vi "GetDnetStrings.vi"() -> ()   [LabVIEW 2011]
uses:
  Controls/Device Cluster.ctl
  <vilib>/Utility/file.llb/Read From Spreadsheet File (string).vi
  GlobalVariables.vi
panel:
  in  "Device Cluster":T1={"Dnet"="", "Node"=0, "Type"="", "ID Number"=0, "SCCM"=0.0, "FullScale"=0.0, "Input Bytes"=0, "Output Bytes"=0, "Input Start Location"=0, "Output Start Location"=0, "Enabled"=TRUE, "Bytes"=[0, 0, 0]}
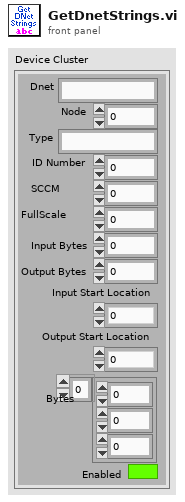
[diagram p1: front panel]
types:
  T1 = typedef "Device Cluster.ctl" = cluster{"Dnet":string, "Node":i32, "Type":string, "ID Number":u8, "SCCM":dbl, "FullScale":dbl, "Input Bytes":i32, "Output Bytes":i32, "Input Start Location":i32, "Output Start Location":i32, "Enabled":bool, "Bytes":u8[]}
  T2 = cluster{"all rows[0]":string, "all rows[1]":string, "all rows[2]":string, "all rows[3]":string, "all rows[4]":string, "all rows[5]":string, "all rows[6]":string, "all rows[7]":string, "all rows[8]":string, "all rows[9]":string}
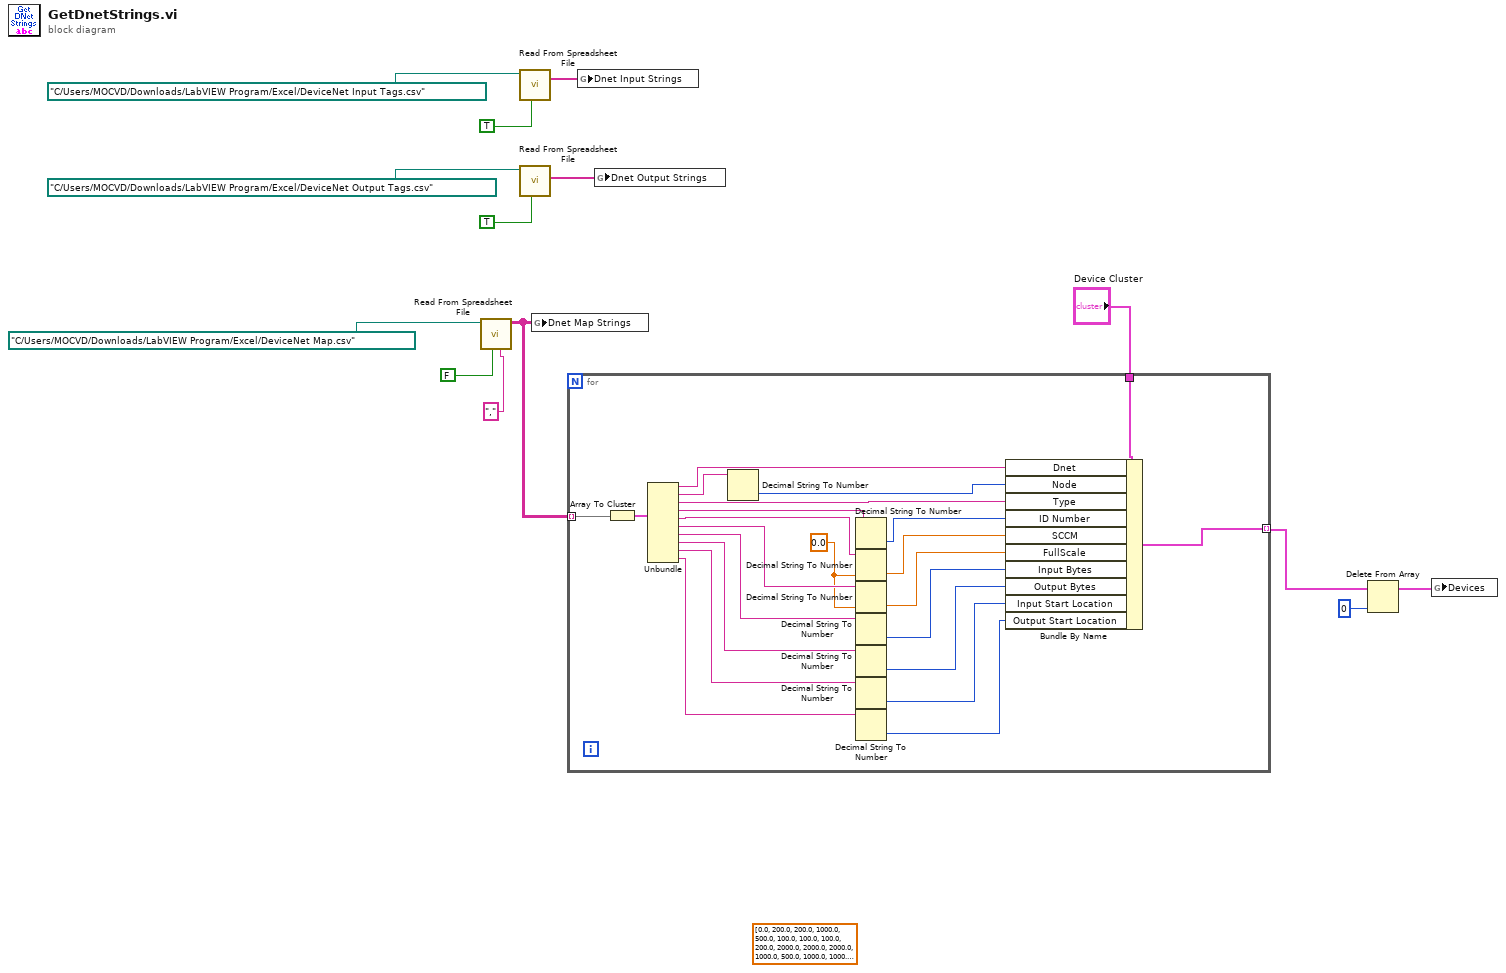
[diagram p0: block diagram]
diagram:
  (unwired) dbl[] [0.0, 200.0, 200.0, 1000.0, 500.0, 100.0, 100.0, 100.0, 200.0, 2000.0, 2000.0, 2000.0, 1000.0, 500.0, 1000.0, 1000.0, 1000.0, 1000.0, 0.0, 1000.0, 100.0, 1000.0, 2000.0, 1000.0, 2000.0, 0.0, 0.0, 5000.0, 5000.0, 5000.0, 5000.0, 0.0, 100.0, 1000.0, 2000.0, 2000.0, 100.0, 100.0, 2000.0, 100.0, 0.0, 10.0, 500.0, 500.0, 2000.0, 200.0, 2000.0, 200.0, 1000.0, 100.0, 1000.0, 100.0, 1000.0, 100.0, 2000.0, 200.0, 500.0, 1000.0, 0.0, 0.0, 0.0, 0.0, 0.0, 0.0, 0.0, 0.0, 0.0, 0.0, 2000.0, 2000.0, 500.0, 0.0, 0.0, 1000.0, 1000.0, 5000.0, 0.0, 0.0, 2000.0, 2000.0, 2000.0, 20000.0, 20000.0, 20000.0, 1000.0, 1000.0, 2000.0]
  n1 = call-poly <vilib>:"Read From Spreadsheet File.vi"("delimiter (\\t)"=",", "transpose (no:F)"=FALSE, "file path (dialog if empty)"=path "C:/Users/MOCVD/Downloads/LabVIEW Program/Excel/DeviceNet Map.csv") -> ("all rows"=w5:string[][])  [unwired: 4 in, 4 out]
  n2 = call-poly <vilib>:"Read From Spreadsheet File.vi"("transpose (no:F)"=TRUE, "file path (dialog if empty)"=path "C:/Users/MOCVD/Downloads/LabVIEW Program/Excel/DeviceNet Input Tags.csv") -> ("first row"=w9:string[])  [unwired: 5 in, 4 out]
  n3 = call-poly <vilib>:"Read From Spreadsheet File.vi"("transpose (no:F)"=TRUE, "file path (dialog if empty)"=path "C:/Users/MOCVD/Downloads/LabVIEW Program/Excel/DeviceNet Output Tags.csv") -> ("first row"=w10:string[])  [unwired: 5 in, 4 out]
  n4 = global write "GlobalVariables.vi" "Dnet Map Strings"(w5) -> ()
  n5 = for {
    tunnel: w5 -> [w37] mode=indexing
    tunnel: "Device Cluster" -> [w35]
    tunnel: [w34] -> w3 mode=indexing
    w19 = 0.0
    n6 = Array To Cluster(array=w37) -> (cluster=w36:T2)
    n7 = Unbundle(w36) -> ("all rows[0]"=w33:string, "all rows[1]"=w31:string, "all rows[2]"=w32:string, "all rows[3]"=w29:string, "all rows[4]"=w22:string, "all rows[5]"=w21:string, "all rows[6]"=w20:string, "all rows[7]"=w23:string, "all rows[8]"=w15:string, "all rows[9]"=w16:string)
    n8 = Decimal String To Number(string=w31) -> (number=w30:i32)  [unwired: 2 in, 1 out]
    n9 = Decimal String To Number(string=w29) -> (number=w28:i32)  [unwired: 2 in, 1 out]
    n10 = Decimal String To Number(string=w22, default (0L)=w19) -> (number=w27:dbl)  [unwired: 1 in, 1 out]
    n11 = Decimal String To Number(string=w21, default (0L)=w19) -> (number=w26:dbl)  [unwired: 1 in, 1 out]
    n12 = Decimal String To Number(string=w20) -> (number=w25:i32)  [unwired: 2 in, 1 out]
    n13 = Decimal String To Number(string=w23) -> (number=w24:i32)  [unwired: 2 in, 1 out]
    n14 = Decimal String To Number(string=w15) -> (number=w18:i32)  [unwired: 2 in, 1 out]
    n15 = Decimal String To Number(string=w16) -> (number=w17:i32)  [unwired: 2 in, 1 out]
    n16 = Bundle By Name(cluster=w35, "Dnet"=w33, "Node"=w30, "Type"=w32, "ID Number"=w28, "SCCM"=w27, "FullScale"=w26, "Input Bytes"=w25, "Output Bytes"=w24, "Input Start Location"=w18, "Output Start Location"=w17) -> (w34:T1)
  }
  n17 = global write "GlobalVariables.vi" "Dnet Input Strings"(w9) -> ()
  n18 = global write "GlobalVariables.vi" "Dnet Output Strings"(w10) -> ()
  n19 = Delete From Array(array=w3, index=0) -> (array with subset deleted=w1:T1[])  [unwired: 1 in, 1 out]
  n20 = global write "GlobalVariables.vi" "Devices"(w1) -> ()
